vi "arrays2.vi"() -> ()   [LabVIEW 2019]
panel:
  out "index of element 2":i32
  out "appended array":bool[](array[boolean])
  in  "OK Button 4":bool
  in  "OK Button 3":bool
  in  "OK Button 2":bool
  in  "OK Button":bool
  in  "element":i32
  out "index of element":i32
  in  "Array":i32[](array[numeric])
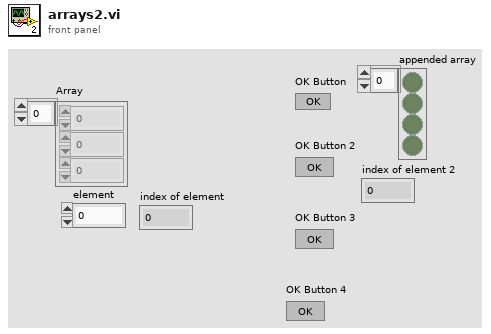
[diagram p1: front panel]
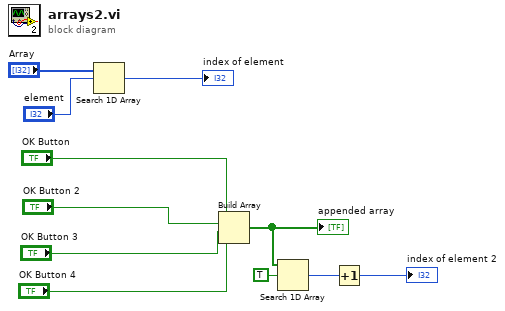
[diagram p0: block diagram]
diagram:
  n1 = Search 1D Array(1D array="Array", element="element") -> (index of element=→"index of element":i32)  [unwired: 1 in]
  n2 = Build Array("OK Button", "OK Button 2", "OK Button 3", "OK Button 4") -> (w4:bool[])
  "appended array" <- w4
  n3 = Search 1D Array(1D array=w4, element=TRUE) -> (index of element=w2:i32)  [unwired: 1 in]
  n4 = Increment(x=w2) -> (x+1=→"index of element 2":i32)
